vi "clear_history.vi"(8 "error in (no error)":errorcluster, 10 "Chat Session Name":string="default", 11 "simple_html_chat_ui in":refnum<class "simple_html_chat_ui.lvclass">) -> (0 "error out":errorcluster, 3 "simple_html_chat_ui out":refnum<class "simple_html_chat_ui.lvclass">)   [LabVIEW 2020, in "simple_html_chat_ui.lvclass"]
uses:
  simple_html_chat_ui.lvclass
  simple_html_chat_ui.lvclass/simple_html_chat_ui.ctl
  <vilib>/httpClient/POSTBuffer.vi
  <vilib>/httpClient/LabVIEWHTTPClient.lvlib
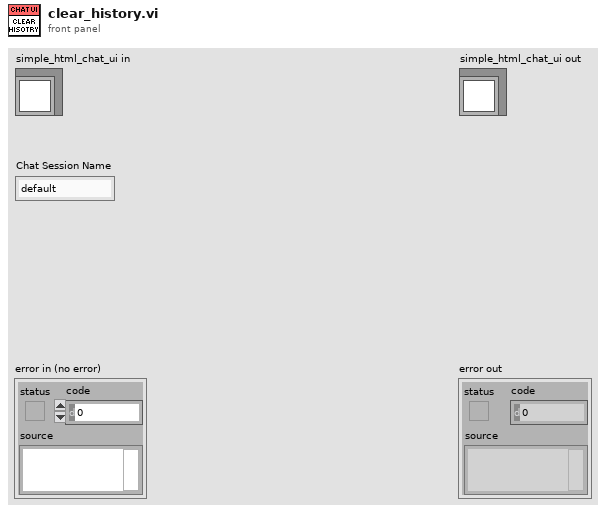
[diagram p1: front panel]
types:
  T1 = typedef "LabVIEWHTTPClient.lvlib/ClientHandle.ctl" = refnum<k1>
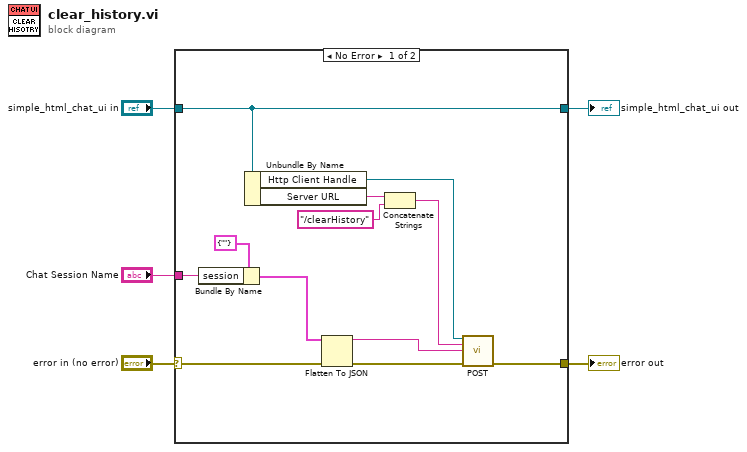
[diagram p0: block diagram]
diagram:
  n1 = case shown="No Error" "error in (no error)" {
    selector: "error in (no error)" -> [w11 w19]
    tunnel: [w10 w19] -> w4
    tunnel: [w9 w18] -> w2
    tunnel: "simple_html_chat_ui in" -> [w9 w18]
    tunnel: "Chat Session Name" -> [w7 _]
    frame No Error {
      n2 = Bundle By Name(cluster=cluster{"session":string} {"session"=""}, "session"=w7) -> (w6:cluster{"session":string})
      n3 = Unbundle By Name(w9) -> ("Http Client Handle"=w14:T1, "Server URL"=w17:string)
      n4 = Flatten To JSON(anything=w6, error in (no error)=w11) -> (JSON string=w12:string, 11:w15:errorcluster)  [unwired: 1 in]
      n5 = Concatenate Strings(w17, "/clearHistory" ("string")) -> (w13:string)
      n6 = call-poly <vilib>:"POST.vi"("client handle"=w14, "url"=w13, "buffer"=w12, "error in (no error)"=w15) -> ("error out"=w10:errorcluster)  [unwired: 8 in, 3 out]
    }
    frame Error {
    }
  }
  "error out" <- w4
  "simple_html_chat_ui out" <- w2
